vi "FipsAdjacent.vi"() -> (11 "Fips":i32[](array[numeric]))   [LabVIEW 2017] (continued)
, MN\"\t27173\t\"Lyon County, MN\"\t27083\n\"Yellow Medicine County, MN\"\t27173\t\"Redwood County, MN\"\t27127\n\"Yellow Medicine County, MN\"\t27173\t\"Renville County, MN\"\t27129\n\"Yellow Medicine County, MN\"\t27173\t\"Yellow Medicine County, MN\"\t27173\n\"Yellow Medicine County, MN\"\t27173\t\"Deuel County, SD\"\t46039\n\"Adams County, MS\"\t28001\t\"Concordia Parish, LA\"\t22029\n\"Adams County, MS\"\t28001\t\"Tensas Parish, LA\"\t22107\n\"Adams County, MS\"\t28001\t\"Adams County, MS\"\t28001\n\"Adams County, MS\"\t28001\t\"Franklin County, MS\"\t28037\n\"Adams County, MS\"\t28001\t\"Jefferson County, MS\"\t28063\n\"Adams County, MS\"\t28001\t\"Wilkinson County, MS\"\t28157\n\"Alcorn County, MS\"\t28003\t\"Alcorn County, MS\"\t28003\n\"Alcorn County, MS\"\t28003\t\"Prentiss County, MS\"\t28117\n\"Alcorn County, MS\"\t28003\t\"Tippah County, MS\"\t28139\n\"Alcorn County, MS\"\t28003\t\"Tishomingo County, MS\"\t28141\n\"Alcorn County, MS\"\t28003\t\"Hardeman County, TN\"\t47069\n\"Alcorn County, MS\"\t28003\t\"Hardin County, TN\"\t47071\n\"Alcorn County, MS\"\t28003\t\"McNairy County, TN\"\t47109\n\"Amite County, MS\"\t28005\t\"East Feliciana Parish, LA\"\t22037\n\"Amite County, MS\"\t28005\t\"St. Helena Parish, LA\"\t22091\n\"Amite County, MS\"\t28005\t\"Tangipahoa Parish, LA\"\t22105\n\"Amite County, MS\"\t28005\t\"Amite County, MS\"\t28005\n\"Amite County, MS\"\t28005\t\"Franklin County, MS\"\t28037\n\"Amite County, MS\"\t28005\t\"Lincoln County, MS\"\t28085\n\"Amite County, MS\"\t28005\t\"Pike County, MS\"\t28113\n\"Amite County, MS\"\t28005\t\"Wilkinson County, MS\"\t28157\n\"Attala County, MS\"\t28007\t\"Attala County, MS\"\t28007\n\"Attala County, MS\"\t28007\t\"Carroll County, MS\"\t28015\n\"Attala County, MS\"\t28007\t\"Choctaw County, MS\"\t28019\n\"Attala County, MS\"\t28007\t\"Holmes County, MS\"\t28051\n\"Attala County, MS\"\t28007\t\"Leake County, MS\"\t28079\n\"Attala County, MS\"\t28007\t\"Madison County, MS\"\t28089\n\"Attala County, MS\"\t28007\t\"Montgomery County, MS\"\t28097\n\"Attala County, MS\"\t28007\t\"Neshoba County, MS\"\t28099\n\"Attala County, MS\"\t28007\t\"Winston County, MS\"\t28159\n\"Attala County, MS\"\t28007\t\"Yazoo County, MS\"\t28163\n\"Benton County, MS\"\t28009\t\"Benton County, MS\"\t28009\n\"Benton County, MS\"\t28009\t\"Marshall County, MS\"\t28093\n\"Benton County, MS\"\t28009\t\"Tippah County, MS\"\t28139\n\"Benton County, MS\"\t28009\t\"Union County, MS\"\t28145\n\"Benton County, MS\"\t28009\t\"Fayette County, TN\"\t47047\n\"Benton County, MS\"\t28009\t\"Hardeman County, TN\"\t47069\n\"Bolivar County, MS\"\t28011\t\"Chicot County, AR\"\t05017\n\"Bolivar County, MS\"\t28011\t\"Desha County, AR\"\t05041\n\"Bolivar County, MS\"\t28011\t\"Phillips County, AR\"\t05107\n\"Bolivar County, MS\"\t28011\t\"Bolivar County, MS\"\t28011\n\"Bolivar County, MS\"\t28011\t\"Coahoma County, MS\"\t28027\n\"Bolivar County, MS\"\t28011\t\"Sunflower County, MS\"\t28133\n\"Bolivar County, MS\"\t28011\t\"Washington County, MS\"\t28151\n\"Calhoun County, MS\"\t28013\t\"Calhoun County, MS\"\t28013\n\"Calhoun County, MS\"\t28013\t\"Chickasaw County, MS\"\t28017\n\"Calhoun County, MS\"\t28013\t\"Grenada County, MS\"\t28043\n\"Calhoun County, MS\"\t28013\t\"Lafayette County, MS\"\t28071\n\"Calhoun County, MS\"\t28013\t\"Pontotoc County, MS\"\t28115\n\"Calhoun County, MS\"\t28013\t\"Webster County, MS\"\t28155\n\"Calhoun County, MS\"\t28013\t\"Yalobusha County, MS\"\t28161\n\"Carroll County, MS\"\t28015\t\"Attala County, MS\"\t28007\n\"Carroll County, MS\"\t28015\t\"Carroll County, MS\"\t28015\n\"Carroll County, MS\"\t28015\t\"Grenada County, MS\"\t28043\n\"Carroll County, MS\"\t28015\t\"Holmes County, MS\"\t28051\n\"Carroll County, MS\"\t28015\t\"Leflore County, MS\"\t28083\n\"Carroll County, MS\"\t28015\t\"Montgomery County, MS\"\t28097\n\"Chickasaw County, MS\"\t28017\t\"Calhoun County, MS\"\t28013\n\"Chickasaw County, MS\"\t28017\t\"Chickasaw County, MS\"\t28017\n\"Chickasaw County, MS\"\t28017\t\"Clay County, MS\"\t28025\n\"Chickasaw County, MS\"\t28017\t\"Lee County, MS\"\t28081\n\"Chickasaw County, MS\"\t28017\t\"Monroe County, MS\"\t28095\n\"Chickasaw County, MS\"\t28017\t\"Pontotoc County, MS\"\t28115\n\"Chickasaw County, MS\"\t28017\t\"Webster County, MS\"\t28155\n\"Choctaw County, MS\"\t28019\t\"Attala County, MS\"\t28007\n\"Choctaw County, MS\"\t28019\t\"Choctaw County, MS\"\t28019\n\"Choctaw County, MS\"\t28019\t\"Montgomery County, MS\"\t28097\n\"Choctaw County, MS\"\t28019\t\"Oktibbeha County, MS\"\t28105\n\"Choctaw County, MS\"\t28019\t\"Webster County, MS\"\t28155\n\"Choctaw County, MS\"\t28019\t\"Winston County, MS\"\t28159\n\"Claiborne County, MS\"\t28021\t\"Tensas Parish, LA\"\t22107\n\"Claiborne County, MS\"\t28021\t\"Claiborne County, MS\"\t28021\n\"Claiborne County, MS\"\t28021\t\"Copiah County, MS\"\t28029\n\"Claiborne County, MS\"\t28021\t\"Hinds County, MS\"\t28049\n\"Claiborne County, MS\"\t28021\t\"Jefferson County, MS\"\t28063\n\"Claiborne County, MS\"\t28021\t\"Warren County, MS\"\t28149\n\"Clarke County, MS\"\t28023\t\"Choctaw County, AL\"\t01023\n\"Clarke County, MS\"\t28023\t\"Clarke County, MS\"\t28023\n\"Clarke County, MS\"\t28023\t\"Jasper County, MS\"\t28061\n\"Clarke County, MS\"\t28023\t\"Lauderdale County, MS\"\t28075\n\"Clarke County, MS\"\t28023\t\"Newton County, MS\"\t28101\n\"Clarke County, MS\"\t28023\t\"Wayne County, MS\"\t28153\n\"Clay County, MS\"\t28025\t\"Chickasaw County, MS\"\t28017\n\"Clay County, MS\"\t28025\t\"Clay County, MS\"\t28025\n\"Clay County, MS\"\t28025\t\"Lowndes County, MS\"\t28087\n\"Clay County, MS\"\t28025\t\"Monroe County, MS\"\t28095\n\"Clay County, MS\"\t28025\t\"Oktibbeha County, MS\"\t28105\n\"Clay County, MS\"\t28025\t\"Webster County, MS\"\t28155\n\"Coahoma County, MS\"\t28027\t\"Phillips County, AR\"\t05107\n\"Coahoma County, MS\"\t28027\t\"Bolivar County, MS\"\t28011\n\"Coahoma County, MS\"\t28027\t\"Coahoma County, MS\"\t28027\n\"Coahoma County, MS\"\t28027\t\"Quitman County, MS\"\t28119\n\"Coahoma County, MS\"\t28027\t\"Sunflower County, MS\"\t28133\n\"Coahoma County, MS\"\t28027\t\"Tallahatchie County, MS\"\t28135\n\"Coahoma County, MS\"\t28027\t\"Tunica County, MS\"\t28143\n\"Copiah County, MS\"\t28029\t\"Claiborne County, MS\"\t28021\n\"Copiah County, MS\"\t28029\t\"Copiah County, MS\"\t28029\n\"Copiah County, MS\"\t28029\t\"Hinds County, MS\"\t28049\n\"Copiah County, MS\"\t28029\t\"Jefferson County, MS\"\t28063\n\"Copiah County, MS\"\t28029\t\"Lawrence County, MS\"\t28077\n\"Copiah County, MS\"\t28029\t\"Lincoln County, MS\"\t28085\n\"Copiah County, MS\"\t28029\t\"Rankin County, MS\"\t28121\n\"Copiah County, MS\"\t28029\t\"Simpson County, MS\"\t28127\n\"Covington County, MS\"\t28031\t\"Covington County, MS\"\t28031\n\"Covington County, MS\"\t28031\t\"Forrest County, MS\"\t28035\n\"Covington County, MS\"\t28031\t\"Jefferson Davis County, MS\"\t28065\n\"Covington County, MS\"\t28031\t\"Jones County, MS\"\t28067\n\"Covington County, MS\"\t28031\t\"Lamar County, MS\"\t28073\n\"Covington County, MS\"\t28031\t\"Simpson County, MS\"\t28127\n\"Covington County, MS\"\t28031\t\"Smith County, MS\"\t28129\n\"DeSoto County, MS\"\t28033\t\"Crittenden County, AR\"\t05035\n\"DeSoto County, MS\"\t28033\t\"DeSoto County, MS\"\t28033\n\"DeSoto County, MS\"\t28033\t\"Marshall County, MS\"\t28093\n\"DeSoto County, MS\"\t28033\t\"Tate County, MS\"\t28137\n\"DeSoto County, MS\"\t28033\t\"Tunica County, MS\"\t28143\n\"DeSoto County, MS\"\t28033\t\"Shelby County, TN\"\t47157\n\"Forrest County, MS\"\t28035\t\"Covington County, MS\"\t28031\n\"Forrest County, MS\"\t28035\t\"Forrest County, MS\"\t28035\n\"Forrest County, MS\"\t28035\t\"Jones County, MS\"\t28067\n\"Forrest County, MS\"\t28035\t\"Lamar County, MS\"\t28073\n\"Forrest County, MS\"\t28035\t\"Pearl River County, MS\"\t28109\n\"Forrest County, MS\"\t28035\t\"Perry County, MS\"\t28111\n\"Forrest County, MS\"\t28035\t\"Stone County, MS\"\t28131\n\"Franklin County, MS\"\t28037\t\"Adams County, MS\"\t28001\n\"Franklin County, MS\"\t28037\t\"Amite County, MS\"\t28005\n\"Franklin County, MS\"\t28037\t\"Franklin County, MS\"\t28037\n\"Franklin County, MS\"\t28037\t\"Jefferson County, MS\"\t28063\n\"Franklin County, MS\"\t28037\t\"Lincoln County, MS\"\t28085\n\"Franklin County, MS\"\t28037\t\"Wilkinson County, MS\"\t28157\n\"George County, MS\"\t28039\t\"Mobile County, AL\"\t01097\n\"George County, MS\"\t28039\t\"George County, MS\"\t28039\n\"George County, MS\"\t28039\t\"Greene County, MS\"\t28041\n\"George County, MS\"\t28039\t\"Jackson County, MS\"\t28059\n\"George County, MS\"\t28039\t\"Perry County, MS\"\t28111\n\"George County, MS\"\t28039\t\"Stone County, MS\"\t28131\n\"Greene County, MS\"\t28041\t\"Mobile County, AL\"\t01097\n\"Greene County, MS\"\t28041\t\"Washington County, AL\"\t01129\n\"Greene County, MS\"\t28041\t\"George County, MS\"\t28039\n\"Greene County, MS\"\t28041\t\"Greene County, MS\"\t28041\n\"Greene County, MS\"\t28041\t\"Perry County, MS\"\t28111\n\"Greene County, MS\"\t28041\t\"Wayne County, MS\"\t28153\n\"Grenada County, MS\"\t28043\t\"Calhoun County, MS\"\t28013\n\"Grenada County, MS\"\t28043\t\"Carroll County, MS\"\t28015\n\"Grenada County, MS\"\t28043\t\"Grenada County, MS\"\t28043\n\"Grenada County, MS\"\t28043\t\"Leflore County, MS\"\t28083\n\"Grenada County, MS\"\t28043\t\"Montgomery County, MS\"\t28097\n\"Grenada County, MS\"\t28043\t\"Tallahatchie County, MS\"\t28135\n\"Grenada County, MS\"\t28043\t\"Webster County, MS\"\t28155\n\"Grenada County, MS\"\t28043\t\"Yalobusha County, MS\"\t28161\n\"Hancock County, MS\"\t28045\t\"St. Bernard Parish, LA\"\t22087\n\"Hancock County, MS\"\t28045\t\"St. Tammany Parish, LA\"\t22103\n\"Hancock County, MS\"\t28045\t\"Hancock County, MS\"\t28045\n\"Hancock County, MS\"\t28045\t\"Harrison County, MS\"\t28047\n\"Hancock County, MS\"\t28045\t\"Pearl River County, MS\"\t28109\n\"Hancock County, MS\"\t28045\t\"Stone County, MS\"\t28131\n\"Harrison County, MS\"\t28047\t\"St. Bernard Parish, LA\"\t22087\n\"Harrison County, MS\"\t28047\t\"Hancock County, MS\"\t28045\n\"Harrison County, MS\"\t28047\t\"Harrison County, MS\"\t28047\n\"Harrison County, MS\"\t28047\t\"Jackson County, MS\"\t28059\n\"Harrison County, MS\"\t28047\t\"Pearl River County, MS\"\t28109\n\"Harrison County, MS\"\t28047\t\"Stone County, MS\"\t28131\n\"Hinds County, MS\"\t28049\t\"Claiborne County, MS\"\t28021\n\"Hinds County, MS\"\t28049\t\"Copiah County, MS\"\t28029\n\"Hinds County, MS\"\t28049\t\"Hinds County, MS\"\t28049\n\"Hinds County, MS\"\t28049\t\"Madison County, MS\"\t28089\n\"Hinds County, MS\"\t28049\t\"Rankin County, MS\"\t28121\n\"Hinds County, MS\"\t28049\t\"Simpson County, MS\"\t28127\n\"Hinds County, MS\"\t28049\t\"Warren County, MS\"\t28149\n\"Hinds County, MS\"\t28049\t\"Yazoo County, MS\"\t28163\n\"Holmes County, MS\"\t28051\t\"Attala County, MS\"\t28007\n\"Holmes County, MS\"\t28051\t\"Carroll County, MS\"\t28015\n\"Holmes County, MS\"\t28051\t\"Holmes County, MS\"\t28051\n\"Holmes County, MS\"\t28051\t\"Humphreys County, MS\"\t28053\n\"Holmes County, MS\"\t28051\t\"Leflore County, MS\"\t28083\n\"Holmes County, MS\"\t28051\t\"Madison County, MS\"\t28089\n\"Holmes County, MS\"\t28051\t\"Yazoo County, MS\"\t28163\n\"Humphreys County, MS\"\t28053\t\"Holmes County, MS\"\t28051\n\"Humphreys County, MS\"\t28053\t\"Humphreys County, MS\"\t28053\n\"Humphreys County, MS\"\t28053\t\"Leflore County, MS\"\t28083\n\"Humphreys County, MS\"\t28053\t\"Sharkey County, MS\"\t28125\n\"Humphreys County, MS\"\t28053\t\"Sunflower County, MS\"\t28133\n\"Humphreys County, MS\"\t28053\t\"Washington County, MS\"\t28151\n\"Humphreys County, MS\"\t28053\t\"Yazoo County, MS\"\t28163\n\"Issaquena County, MS\"\t28055\t\"Chicot County, AR\"\t05017\n\"Issaquena County, MS\"\t28055\t\"East Carroll Parish, LA\"\t22035\n\"Issaquena County, MS\"\t28055\t\"Issaquena County, MS\"\t28055\n\"Issaquena County, MS\"\t28055\t\"Sharkey County, MS\"\t28125\n\"Issaquena County, MS\"\t28055\t\"Warren County, MS\"\t28149\n\"Issaquena County, MS\"\t28055\t\"Washington County, MS\"\t28151\n\"Issaquena County, MS\"\t28055\t\"Yazoo County, MS\"\t28163\n\"Itawamba County, MS\"\t28057\t\"Franklin County, AL\"\t01059\n\"Itawamba County, MS\"\t28057\t\"Marion County, AL\"\t01093\n\"Itawamba County, MS\"\t28057\t\"Itawamba County, MS\"\t28057\n\"Itawamba County, MS\"\t28057\t\"Lee County, MS\"\t28081\n\"Itawamba County, MS\"\t28057\t\"Monroe County, MS\"\t28095\n\"Itawamba County, MS\"\t28057\t\"Prentiss County, MS\"\t28117\n\"Itawamba County, MS\"\t28057\t\"Tishomingo County, MS\"\t28141\n\"Jackson County, MS\"\t28059\t\"Mobile County, AL\"\t01097\n\"Jackson County, MS\"\t28059\t\"George County, MS\"\t28039\n\"Jackson County, MS\"\t28059\t\"Harrison County, MS\"\t28047\n\"Jackson County, MS\"\t28059\t\"Jackson County, MS\"\t28059\n\"Jackson County, MS\"\t28059\t\"Stone County, MS\"\t28131\n\"Jasper County, MS\"\t28061\t\"Clarke County, MS\"\t28023\n\"Jasper County, MS\"\t28061\t\"Jasper County, MS\"\t28061\n\"Jasper County, MS\"\t28061\t\"Jones County, MS\"\t28067\n\"Jasper County, MS\"\t28061\t\"Lauderdale County, MS\"\t28075\n\"Jasper County, MS\"\t28061\t\"Newton County, MS\"\t28101\n\"Jasper County, MS\"\t28061\t\"Scott County, MS\"\t28123\n\"Jasper County, MS\"\t28061\t\"Smith County, MS\"\t28129\n\"Jasper County, MS\"\t28061\t\"Wayne County, MS\"\t28153\n\"Jefferson County, MS\"\t28063\t\"Tensas Parish, LA\"\t22107\n\"Jefferson County, MS\"\t28063\t\"Adams County, MS\"\t28001\n\"Jefferson County, MS\"\t28063\t\"Claiborne County, MS\"\t28021\n\"Jefferson County, MS\"\t28063\t\"Copiah County, MS\"\t28029\n\"Jefferson County, MS\"\t28063\t\"Franklin County, MS\"\t28037\n\"Jefferson County, MS\"\t28063\t\"Jefferson County, MS\"\t28063\n\"Jefferson County, MS\"\t28063\t\"Lincoln County, MS\"\t28085\n\"Jefferson Davis County, MS\"\t28065\t\"Covington County, MS\"\t28031\n\"Jefferson Davis County, MS\"\t28065\t\"Jefferson Davis County, MS\"\t28065\n\"Jefferson Davis County, MS\"\t28065\t\"Lamar County, MS\"\t28073\n\"Jefferson Davis County, MS\"\t28065\t\"Lawrence County, MS\"\t28077\n\"Jefferson Davis County, MS\"\t28065\t\"Marion County, MS\"\t28091\n\"Jefferson Davis County, MS\"\t28065\t\"Simpson County, MS\"\t28127\n\"Jones County, MS\"\t28067\t\"Covington County, MS\"\t28031\n\"Jones County, MS\"\t28067\t\"Forrest County, MS\"\t28035\n\"Jones County, MS\"\t28067\t\"Jasper County, MS\"\t28061\n\"Jones County, MS\"\t28067\t\"Jones County, MS\"\t28067\n\"Jones County, MS\"\t28067\t\"Perry County, MS\"\t28111\n\"Jones County, MS\"\t28067\t\"Smith County, MS\"\t28129\n\"Jones County, MS\"\t28067\t\"Wayne County, MS\"\t28153\n\"Kemper County, MS\"\t28069\t\"Sumter County, AL\"\t01119\n\"Kemper County, MS\"\t28069\t\"Kemper County, MS\"\t28069\n\"Kemper County, MS\"\t28069\t\"Lauderdale County, MS\"\t28075\n\"Kemper County, MS\"\t28069\t\"Neshoba County, MS\"\t28099\n\"Kemper County, MS\"\t28069\t\"Newton County, MS\"\t28101\n\"Kemper County, MS\"\t28069\t\"Noxubee County, MS\"\t28103\n\"Kemper County, MS\"\t28069\t\"Winston County, MS\"\t28159\n\"Lafayette County, MS\"\t28071\t\"Calhoun County, MS\"\t28013\n\"Lafayette County, MS\"\t28071\t\"Lafayette County, MS\"\t28071\n\"Lafayette County, MS\"\t28071\t\"Marshall County, MS\"\t28093\n\"Lafayette County, MS\"\t28071\t\"Panola County, MS\"\t28107\n\"Lafayette County, MS\"\t28071\t\"Pontotoc County, MS\"\t28115\n\"Lafayette County, MS\"\t28071\t\"Tate County, MS\"\t28137\n\"Lafayette County, MS\"\t28071\t\"Union County, MS\"\t28145\n\"Lafayette County, MS\"\t28071\t\"Yalobusha County, MS\"\t28161\n\"Lamar County, MS\"\t28073\t\"Covington County, MS\"\t28031\n\"Lamar County, MS\"\t28073\t\"Forrest County, MS\"\t28035\n\"Lamar County, MS\"\t28073\t\"Jefferson Davis County, MS\"\t28065\n\"Lamar County, MS\"\t28073\t\"Lamar County, MS\"\t28073\n\"Lamar County, MS\"\t28073\t\"Marion County, MS\"\t28091\n\"Lamar County, MS\"\t28073\t\"Pearl River County, MS\"\t28109\n\"Lauderdale County, MS\"\t28075\t\"Choctaw County, AL\"\t01023\n\"Lauderdale County, MS\"\t28075\t\"Sumter County, AL\"\t01119\n\"Lauderdale County, MS\"\t28075\t\"Clarke County, MS\"\t28023\n\"Lauderdale County, MS\"\t28075\t\"Jasper County, MS\"\t28061\n\"Lauderdale County, MS\"\t28075\t\"Kemper County, MS\"\t28069\n\"Lauderdale County, MS\"\t28075\t\"Lauderdale County, MS\"\t28075\n\"Lauderdale County, MS\"\t28075\t\"Neshoba County, MS\"\t28099\n\"Lauderdale County, MS\"\t28075\t\"Newton County, MS\"\t28101\n\"Lawrence County, MS\"\t28077\t\"Copiah County, MS\"\t28029\n\"Lawrence County, MS\"\t28077\t\"Jefferson Davis County, MS\"\t28065\n\"Lawrence County, MS\"\t28077\t\"Lawrence County, MS\"\t28077\n\"Lawrence County, MS\"\t28077\t\"Lincoln County, MS\"\t28085\n\"Lawrence County, MS\"\t28077\t\"Marion County, MS\"\t28091\n\"Lawrence County, MS\"\t28077\t\"Simpson County, MS\"\t28127\n\"Lawrence County, MS\"\t28077\t\"Walthall County, MS\"\t28147\n\"Leake County, MS\"\t28079\t\"Attala County, MS\"\t28007\n\"Leake County, MS\"\t28079\t\"Leake County, MS\"\t28079\n\"Leake County, MS\"\t28079\t\"Madison County, MS\"\t28089\n\"Leake County, MS\"\t28079\t\"Neshoba County, MS\"\t28099\n\"Leake County, MS\"\t28079\t\"Newton County, MS\"\t28101\n\"Leake County, MS\"\t28079\t\"Scott County, MS\"\t28123\n\"Leake County, MS\"\t28079\t\"Winston County, MS\"\t28159\n\"Lee County, MS\"\t28081\t\"Chickasaw County, MS\"\t28017\n\"Lee County, MS\"\t28081\t\"Itawamba County, MS\"\t28057\n\"Lee County, MS\"\t28081\t\"Lee County, MS\"\t28081\n\"Lee County, MS\"\t28081\t\"Monroe County, MS\"\t28095\n\"Lee County, MS\"\t28081\t\"Pontotoc County, MS\"\t28115\n\"Lee County, MS\"\t28081\t\"Prentiss County, MS\"\t28117\n\"Lee County, MS\"\t28081\t\"Union County, MS\"\t28145\n\"Leflore County, MS\"\t28083\t\"Carroll County, MS\"\t28015\n\"Leflore County, MS\"\t28083\t\"Grenada County, MS\"\t28043\n\"Leflore County, MS\"\t28083\t\"Holmes County, MS\"\t28051\n\"Leflore County, MS\"\t28083\t\"Humphreys County, MS\"\t28053\n\"Leflore County, MS\"\t28083\t\"Leflore County, MS\"\t28083\n\"Leflore County, MS\"\t28083\t\"Sunflower County, MS\"\t28133\n\"Leflore County, MS\"\t28083\t\"Tallahatchie County, MS\"\t28135\n\"Lincoln County, MS\"\t28085\t\"Amite County, MS\"\t28005\n\"Lincoln County, MS\"\t28085\t\"Copiah County, MS\"\t28029\n\"Lincoln County, MS\"\t28085\t\"Franklin County, MS\"\t28037\n\"Lincoln County, MS\"\t28085\t\"Jefferson County, MS\"\t28063\n\"Lincoln County, MS\"\t28085\t\"Lawrence County, MS\"\t28077\n\"Lincoln County, MS\"\t28085\t\"Lincoln County, MS\"\t28085\n\"Lincoln County, MS\"\t28085\t\"Pike County, MS\"\t28113\n\"Lincoln County, MS\"\t28085\t\"Walthall County, MS\"\t28147\n\"Lowndes County, MS\"\t28087\t\"Lamar County, AL\"\t01075\n\"Lowndes County, MS\"\t28087\t\"Pickens County, AL\"\t01107\n\"Lowndes County, MS\"\t28087\t\"Clay County, MS\"\t28025\n\"Lowndes County, MS\"\t28087\t\"Lowndes County, MS\"\t28087\n\"Lowndes County, MS\"\t28087\t\"Monroe County, MS\"\t28095\n\"Lowndes County, MS\"\t28087\t\"Noxubee County, MS\"\t28103\n\"Lowndes County, MS\"\t28087\t\"Oktibbeha County, MS\"\t28105\n\"Madison County, MS\"\t28089\t\"Attala County, MS\"\t28007\n\"Madison County, MS\"\t28089\t\"Hinds County, MS\"\t28049\n\"Madison County, MS\"\t28089\t\"Holmes County, MS\"\t28051\n\"Madison County, MS\"\t28089\t\"Leake County, MS\"\t28079\n\"Madison County, MS\"\t28089\t\"Madison County, MS\"\t28089\n\"Madison County, MS\"\t28089\t\"Rankin County, MS\"\t28121\n\"Madison County, MS\"\t28089\t\"Scott County, MS\"\t28123\n\"Madison County, MS\"\t28089\t\"Yazoo County, MS\"\t28163\n\"Marion County, MS\"\t28091\t\"Washington Parish, LA\"\t22117\n\"Marion County, MS\"\t28091\t\"Jefferson Davis County, MS\"\t28065\n\"Marion County, MS\"\t28091\t\"Lamar County, MS\"\t28073\n\"Marion County, MS\"\t28091\t\"Lawrence County, MS\"\t28077\n\"Marion County, MS\"\t28091\t\"Marion County, MS\"\t28091\n\"Marion County, MS\"\t28091\t\"Pearl River County, MS\"\t28109\n\"Marion County, MS\"\t28091\t\"Walthall County, MS\"\t28147\n\"Marshall County, MS\"\t28093\t\"Benton County, MS\"\t28009\n\"Marshall County, MS\"\t28093\t\"DeSoto County, MS\"\t28033\n\"Marshall County, MS\"\t28093\t\"Lafayette County, MS\"\t28071\n\"Marshall County, MS\"\t28093\t\"Marshall County, MS\"\t28093\n\"Marshall County, MS\"\t28093\t\"Tate County, MS\"\t28137\n\"Marshall County, MS\"\t28093\t\"Union County, MS\"\t28145\n\"Marshall County, MS\"\t28093\t\"Fayette County, TN\"\t47047\n\"Marshall County, MS\"\t28093\t\"Shelby County, TN\"\t47157\n\"Monroe County, MS\"\t28095\t\"Lamar County, AL\"\t01075\n\"Monroe County, MS\"\t28095\t\"Marion County, AL\"\t01093\n\"Monroe County, MS\"\t28095\t\"Chickasaw County, MS\"\t28017\n\"Monroe County, MS\"\t28095\t\"Clay County, MS\"\t28025\n\"Monroe County, MS\"\t28095\t\"Itawamba County, MS\"\t28057\n\"Monroe County, MS\"\t28095\t\"Lee County, MS\"\t28081\n\"Monroe County, MS\"\t28095\t\"Lowndes County, MS\"\t28087\n\"Monroe County, MS\"\t28095\t\"Monroe County, MS\"\t28095\n\"Montgomery County, MS\"\t28097\t\"Attala County, MS\"\t28007\n\"Montgomery County, MS\"\t28097\t\"Carroll County, MS\"\t28015\n\"Montgomery County, MS\"\t28097\t\"Choctaw County, MS\"\t28019\n\"Montgomery County, MS\"\t28097\t\"Grenada County, MS\"\t28043\n\"Montgomery County, MS\"\t28097\t\"Montgomery County, MS\"\t28097\n\"Montgomery County, MS\"\t28097\t\"Webster County, MS\"\t28155\n\"Neshoba County, MS\"\t28099\t\"Attala County, MS\"\t28007\n\"Neshoba County, MS\"\t28099\t\"Kemper County, MS\"\t28069\n\"Neshoba County, MS\"\t28099\t\"Lauderdale County, MS\"\t28075\n\"Neshoba County, MS\"\t28099\t\"Leake County, MS\"\t28079\n\"Neshoba County, MS\"\t28099\t\"Neshoba County, MS\"\t28099\n\"Neshoba County, MS\"\t28099\t\"Newton County, MS\"\t28101\n\"Neshoba County, MS\"\t28099\t\"Winston County, MS\"\t28159\n\"Newton County, MS\"\t28101\t\"Clarke County, MS\"\t28023\n\"Newton County, MS\"\t28101\t\"Jasper County, MS\"\t28061\n\"Newton County, MS\"\t28101\t\"Kemper County, MS\"\t28069\n\"Newton County, MS\"\t28101\t\"Lauderdale County, MS\"\t28075\n\"Newton County, MS\"\t28101\t\"Leake County, MS\"\t28079\n\"Newton County, MS\"\t28101\t\"Neshoba County, MS\"\t28099\n\"Newton County, MS\"\t28101\t\"Newton County, MS\"\t28101\n\"Newton County, MS\"\t28101\t\"Scott County, MS\"\t28123\n\"Newton County, MS\"\t28101\t\"Smith County, MS\"\t28129\n\"Noxubee County, MS\"\t28103\t\"Pickens County, AL\"\t01107\n\"Noxubee County, MS\"\t28103\t\"Sumter County, AL\"\t01119\n\"Noxubee County, MS\"\t28103\t\"Kemper County, MS\"\t28069\n\"Noxubee County, MS\"\t28103\t\"Lowndes County, MS\"\t28087\n\"Noxubee County, MS\"\t28103\t\"Noxubee County, MS\"\t28103\n\"Noxubee County, MS\"\t28103\t\"Oktibbeha County, MS\"\t28105\n\"Noxubee County, MS\"\t28103\t\"Winston County, MS\"\t28159\n\"Oktibbeha County, MS\"\t28105\t\"Choctaw County, MS\"\t28019\n\"Oktibbeha County, MS\"\t28105\t\"Clay County, MS\"\t28025\n\"Oktibbeha County, MS\"\t28105\t\"Lowndes County, MS\"\t28087\n\"Oktibbeha County, MS\"\t28105\t\"Noxubee County, MS\"\t28103\n\"Oktibbeha County, MS\"\t28105\t\"Oktibbeha County, MS\"\t28105\n\"Oktibbeha County, MS\"\t28105\t\"Webster County, MS\"\t28155\n\"Oktibbeha County, MS\"\t28105\t\"Winston County, MS\"\t28159\n\"Panola County, MS\"\t28107\t\"Lafayette County, MS\"\t28071\n\"Panola County, MS\"\t28107\t\"Panola County, MS\"\t28107\n\"Panola County, MS\"\t28107\t\"Quitman County, MS\"\t28119\n\"Panola County, MS\"\t28107\t\"Tallahatchie County, MS\"\t28135\n\"Panola County, MS\"\t28107\t\"Tate County, MS\"\t28137\n\"Panola County, MS\"\t28107\t\"Tunica County, MS\"\t28143\n\"Panola County, MS\"\t28107\t\"Yalobusha County, MS\"\t28161\n\"Pearl River County, MS\"\t28109\t\"St. Tammany Parish, LA\"\t22103\n\"Pearl River County, MS\"\t28109\t\"Washington Parish, LA\"\t22117\n\"Pearl River County, MS\"\t28109\t\"Forrest County, MS\"\t28035\n\"Pearl River County, MS\"\t28109\t\"Hancock County, MS\"\t28045\n\"Pearl River County, MS\"\t28109\t\"Harrison County, MS\"\t28047\n\"Pearl River County, MS\"\t28109\t\"Lamar County, MS\"\t28073\n\"Pearl River County, MS\"\t28109\t\"Marion County, MS\"\t28091\n\"Pearl River County, MS\"\t28109\t\"Pearl River County, MS\"\t28109\n\"Pearl River County, MS\"\t28109\t\"Stone County, MS\"\t28131\n\"Perry County, MS\"\t28111\t\"Forrest County, MS\"\t28035\n\"Perry County, MS\"\t28111\t\"George County, MS\"\t28039\n\"Perry County, MS\"\t28111\t\"Greene County, MS\"\t28041\n\"Perry County, MS\"\t28111\t\"Jones County, MS\"\t28067\n\"Perry County, MS\"\t28111\t\"Perry County, MS\"\t28111\n\"Perry County, MS\"\t28111\t\"Stone County, MS\"\t28131\n\"Perry County, MS\"\t28111\t\"Wayne County, MS\"\t28153\n\"Pike County, MS\"\t28113\t\"Tangipahoa Parish, LA\"\t22105\n\"Pike County, MS\"\t28113\t\"Washington Parish, LA\"\t22117\n\"Pike County, MS\"\t28113\t\"Amite County, MS\"\t28005\n\"Pike County, MS\"\t28113\t\"Lincoln County, MS\"\t28085\n\"Pike County, MS\"\t28113\t\"Pike County, MS\"\t28113\n\"Pike County, MS\"\t28113\t\"Walthall County, MS\"\t28147\n\"Pontotoc County, MS\"\t28115\t\"Calhoun County, MS\"\t28013\n\"Pontotoc County, MS\"\t28115\t\"Chickasaw County, MS\"\t28017\n\"Pontotoc County, MS\"\t28115\t\"Lafayette County, MS\"\t28071\n\"Pontotoc County, MS\"\t28115\t\"Lee County, MS\"\t28081\n\"Pontotoc County, MS\"\t28115\t\"Pontotoc County, MS\"\t28115\n\"Pontotoc County, MS\"\t28115\t\"Union County, MS\"\t28145\n\"Prentiss County, MS\"\t28117\t\"Alcorn County, MS\"\t28003\n\"Prentiss County, MS\"\t28117\t\"Itawamba County, MS\"\t28057\n\"Prentiss County, MS\"\t28117\t\"Lee County, MS\"\t28081\n\"Prentiss County, MS\"\t28117\t\"Prentiss County, MS\"\t28117\n\"Prentiss County, MS\"\t28117\t\"Tippah County, MS\"\t28139\n\"Prentiss County, MS\"\t28117\t\"Tishomingo County, MS\"\t28141\n\"Prentiss County, MS\"\t28117\t\"Union County, MS\"\t28145\n\"Quitman County, MS\"\t28119\t\"Coahoma County, MS\"\t28027\n\"Quitman County, MS\"\t28119\t\"Panola County, MS\"\t28107\n\"Quitman County, MS\"\t28119\t\"Quitman County, MS\"\t28119\n\"Quitman County, MS\"\t28119\t\"Tallahatchie County, MS\"\t28135\n\"Quitman County, MS\"\t28119\t\"Tunica County, MS\"\t28143\n\"Rankin County, MS\"\t28121\t\"Copiah County, MS\"\t28029\n\"Rankin County, MS\"\t28121\t\"Hinds County, MS\"\t28049\n\"Rankin County, MS\"\t28121\t\"Madison County, MS\"\t28089\n\"Rankin County, MS\"\t28121\t\"Rankin County, MS\"\t28121\n\"Rankin County, MS\"\t28121\t\"Scott County, MS\"\t28123\n\"Rankin County, MS\"\t28121\t\"Simpson County, MS\"\t28127\n\"Rankin County, MS\"\t28121\t\"Smith County, MS\"\t28129\n\"Scott County, MS\"\t28123\t\"Jasper County, MS\"\t28061\n\"Scott County, MS\"\t28123\t\"Leake County, MS\"\t28079\n\"Scott County, MS\"\t28123\t\"Madison County, MS\"\t28089\n\"Scott County, MS\"\t28123\t\"Newton County, MS\"\t28101\n\"Scott County, MS\"\t28123\t\"Rankin County, MS\"\t28121\n\"Scott County, MS\"\t28123\t\"Scott County, MS\"\t28123\n\"Scott County, MS\"\t28123\t\"Smith County, MS\"\t28129\n\"Sharkey County, MS\"\t28125\t\"Humphreys County, MS\"\t28053\n\"Sharkey County, MS\"\t28125\t\"Issaquena County, MS\"\t28055\n\"Sharkey County, MS\"\t28125\t\"Sharkey County, MS\"\t28125\n\"Sharkey County, MS\"\t28125\t\"Washington County, MS\"\t28151\n\"Sharkey County, MS\"\t28125\t\"Yazoo County, MS\"\t28163\n\"Simpson County, MS\"\t28127\t\"Copiah County, MS\"\t28029\n\"Simpson County, MS\"\t28127\t\"Covington County, MS\"\t28031\n\"Simpson County, MS\"\t28127\t\"Hinds County, MS\"\t28049\n\"Simpson County, MS\"\t28127\t\"Jefferson Davis County, MS\"\t28065\n\"Simpson County, MS\"\t28127\t\"Lawrence County, MS\"\t28077\n\"Simpson County, MS\"\t28127\t\"Rankin County, MS\"\t28121\n\"Simpson County, MS\"\t28127\t\"Simpson County, MS\"\t28127\n\"Simpson County, MS\"\t28127\t\"Smith County, MS\"\t28129\n\"Smith County, MS\"\t28129\t\"Covington County, MS\"\t28031\n\"Smith County, MS\"\t28129\t\"Jasper County, MS\"\t28061\n\"Smith County, MS\"\t28129\t\"Jones County, MS\"\t28067\n\"Smith County, MS\"\t28129\t\"Newton County, MS\"\t28101\n\"Smith County, MS\"\t28129\t\"Rankin County, MS\"\t28121\n\"Smith County, MS\"\t28129\t\"Scott County, MS\"\t28123\n\"Smith County, MS\"\t28129\t\"Simpson County, MS\"\t28127\n\"Smith County, MS\"\t28129\t\"Smith County, MS\"\t28129\n\"Stone County, MS\"\t28131\t\"Forrest County, MS\"\t28035\n\"Stone County, MS\"\t28131\t\"George County, MS\"\t28039\n\"Stone County, MS\"\t28131\t\"Hancock County, MS\"\t28045\n\"Stone County, MS\"\t28131\t\"Harrison County, MS\"\t28047\n\"Stone County, MS\"\t28131\t\"Jackson County, MS\"\t28059\n\"Stone County, MS\"\t28131\t\"Pearl River County, MS\"\t28109\n\"Stone County, MS\"\t28131\t\"Perry County, MS\"\t28111\n\"Stone County, MS\"\t28131\t\"Stone County, MS\"\t28131\n\"Sunflower County, MS\"\t28133\t\"Bolivar County, MS\"\t28011\n\"Sunflower County, MS\"\t28133\t\"Coahoma County, MS\"\t28027\n\"Sunflower County, MS\"\t28133\t\"Humphreys County, MS\"\t28053\n\"Sunflower County, MS\"\t28133\t\"Leflore County, MS\"\t28083\n\"Sunflower County, MS\"\t28133\t\"Sunflower County, MS\"\t28133\n\"Sunflower County, MS\"\t28133\t\"Tallahatchie County, MS\"\t28135\n\"Sunflower County, MS\"\t28133\t\"Washington County, MS\"\t28151\n\"Tallahatchie County, MS\"\t28135\t\"Coahoma County, MS\"\t28027\n\"Tallahatchie County, MS\"\t28135\t\"Grenada County, MS\"\t28043\n\"Tallahatchie County, MS\"\t28135\t\"Leflore County, MS\"\t28083\n\"Tallahatchie County, MS\"\t28135\t\"Panola County, MS\"\t28107\n\"Tallahatchie County, MS\"\t28135\t\"Quitman County, MS\"\t28119\n\"Tallahatchie County, MS\"\t28135\t\"Sunflower County, MS\"\t28133\n\"Tallahatchie County, MS\"\t28135\t\"Tallahatchie County, MS\"\t28135\n\"Tallahatchie County, MS\"\t28135\t\"Yalobusha County, MS\"\t28161\n\"Tate County, MS\"\t28137\t\"DeSoto County, MS\"\t28033\n\"Tate County, MS\"\t28137\t\"Lafayette County, MS\"\t28071\n\"Tate County, MS\"\t28137\t\"Marshall County, MS\"\t28093\n\"Tate County, MS\"\t28137\t\"Panola County, MS\"\t28107\n\"Tate County, MS\"\t28137\t\"Tate County, MS\"\t28137\n\"Tate County, MS\"\t28137\t\"Tunica County, MS\"\t28143\n\"Tippah County, MS\"\t28139\t\"Alcorn County, MS\"\t28003\n\"Tippah County, MS\"\t28139\t\"Benton County, MS\"\t28009\n\"Tippah County, MS\"\t28139\t\"Prentiss County, MS\"\t28117\n\"Tippah County, MS\"\t28139\t\"Tippah County, MS\"\t28139\n\"Tippah County, MS\"\t28139\t\"Union County, MS\"\t28145\n\"Tippah County, MS\"\t28139\t\"Hardeman County, TN\"\t47069\n\"Tishomingo County, MS\"\t28141\t\"Colbert County, AL\"\t01033\n\"Tishomingo County, MS\"\t28141\t\"Franklin County, AL\"\t01059\n\"Tishomingo County, MS\"\t28141\t\"Lauderdale County, AL\"\t01077\n\"Tishomingo County, MS\"\t28141\t\"Alcorn County, MS\"\t28003\n\"Tishomingo County, MS\"\t28141\t\"Itawamba County, MS\"\t28057\n\"Tishomingo County, MS\"\t28141\t\"Prentiss County, MS\"\t28117\n\"Tishomingo County, MS\"\t28141\t\"Tishomingo County, MS\"\t28141\n\"Tishomingo County, MS\"\t28141\t\"Hardin County, TN\"\t47071\n\"Tunica County, MS\"\t28143\t\"Crittenden County, AR\"\t05035\n\"Tunica County, MS\"\t28143\t\"Lee County, AR\"\t05077\n\"Tunica County, MS\"\t28143\t\"Phillips County, AR\"\t05107\n\"Tunica County, MS\"\t28143\t\"Coahoma County, MS\"\t28027\n\"Tunica County, MS\"\t28143\t\"DeSoto County, MS\"\t28033\n\"Tunica County, MS\"\t28143\t\"Panola County, MS\"\t28107\n\"Tunica County, MS\"\t28143\t\"Quitman County, MS\"\t28119\n\"Tunica County, MS\"\t28143\t\"Tate County, MS\"\t28137\n\"Tunica County, MS\"\t28143\t\"Tunica County, MS\"\t28143\n\"Union County, MS\"\t28145\t\"Benton County, MS\"\t28009\n\"Union County, MS\"\t28145\t\"Lafayette County, MS\"\t28071\n\"Union County, MS\"\t28145\t\"Lee County, MS\"\t28081\n\"Union County, MS\"\t28145\t\"Marshall County, MS\"\t28093\n\"Union County, MS\"\t28145\t\"Pontotoc County, MS\"\t28115\n\"Union County, MS\"\t28145\t\"Prentiss County, MS\"\t28117\n\"Union County, MS\"\t28145\t\"Tippah County, MS\"\t28139\n\"Union County, MS\"\t28145\t\"Union County, MS\"\t28145\n\"Walthall County, MS\"\t28147\t\"Washington Parish, LA\"\t22117\n\"Walthall County, MS\"\t28147\t\"Lawrence County, MS\"\t28077\n\"Walthall County, MS\"\t28147\t\"Lincoln County, MS\"\t28085\n\"Walthall County, MS\"\t28147\t\"Marion County, MS\"\t28091\n\"Walthall County, MS\"\t28147\t\"Pike County, MS\"\t28113\n\"Walthall County, MS\"\t28147\t\"Walthall County, MS\"\t28147\n\"Warren County, MS\"\t28149\t\"East Carroll Parish, LA\"\t22035\n\"Warren County, MS\"\t28149\t\"Madison Parish, LA\"\t22065\n\"Warren County, MS\"\t28149\t\"Tensas Parish, LA\"\t22107\n\"Warren County, MS\"\t28149\t\"Claiborne County, MS\"\t28021\n\"Warren County, MS\"\t28149\t\"Hinds County, MS\"\t28049\n\"Warren County, MS\"\t28149\t\"Issaquena County, MS\"\t28055\n\"Warren County, MS\"\t28149\t\"Warren County, MS\"\t28149\n\"Warren County, MS\"\t28149\t\"Yazoo County, MS\"\t28163\n\"Washington County, MS\"\t28151\t\"Chicot County, AR\"\t05017\n\"Washington County, MS\"\t28151\t\"Bolivar County, MS\"\t28011\n\"Washington County, MS\"\t28151\t\"Humphreys County, MS\"\t28053\n\"Washington County, MS\"\t28151\t\"Issaquena County, MS\"\t28055\n\"Washington County, MS\"\t28151\t\"Sharkey County, MS\"\t28125\n\"Washington County, MS\"\t28151\t\"Sunflower County, MS\"\t28133\n\"Washington County, MS\"\t28151\t\"Washington County, MS\"\t28151\n\"Wayne County, MS\"\t28153\t\"Choctaw County, AL\"\t01023\n\"Wayne County, MS\"\t28153\t\"Washington County, AL\"\t01129\n\"Wayne County, MS\"\t28153\t\"Clarke County, MS\"\t28023\n\"Wayne County, MS\"\t28153\t\"Greene County, MS\"\t28041\n\"Wayne County, MS\"\t28153\t\"Jasper County, MS\"\t28061\n\"Wayne County, MS\"\t28153\t\"Jones County, MS\"\t28067\n\"Wayne County, MS\"\t28153\t\"Perry County, MS\"\t28111\n\"Wayne County, MS\"\t28153\t\"Wayne County, MS\"\t28153\n\"Webster County, MS\"\t28155\t\"Calhoun County, MS\"\t28013\n\"Webster County, MS\"\t28155\t\"Chickasaw County, MS\"\t28017\n\"Webster County, MS\"\t28155\t\"Choctaw County, MS\"\t28019\n\"Webster County, MS\"\t28155\t\"Clay County, MS\"\t28025\n\"Webster County, MS\"\t28155\t\"Grenada County, MS\"\t28043\n\"Webster County, MS\"\t28155\t\"Montgomery County, MS\"\t28097\n\"Webster County, MS\"\t28155\t\"Oktibbeha County, MS\"\t28105\n\"Webster County, MS\"\t28155\t\"Webster County, MS\"\t28155\n\"Wilkinson County, MS\"\t28157\t\"Concordia Parish, LA\"\t22029\n\"Wilkinson County, MS\"\t28157\t\"East Feliciana Parish, LA\"\t22037\n\"Wilkinson County, MS\"\t28157\t\"West Feliciana Parish, LA\"\t22125\n\"Wilkinson County, MS\"\t28157\t\"Adams County, MS\"\t28001\n\"Wilkinson County, MS\"\t28157\t\"Amite County, MS\"\t28005\n\"Wilkinson County, MS\"\t28157\t\"Franklin County, MS\"\t28037\n\"Wilkinson County, MS\"\t28157\t\"Wilkinson County, MS\"\t28157\n\"Winston County, MS\"\t28159\t\"Attala County, MS\"\t28007\n\"Winston County, MS\"\t28159\t\"Choctaw County, MS\"\t28019\n\"Winston County, MS\"\t28159\t\"Kemper County, MS\"\t28069\n\"Winston County, MS\"\t28159\t\"Leake County, MS\"\t28079\n\"Winston County, MS\"\t28159\t\"Neshoba County, MS\"\t28099\n\"Winston County, MS\"\t28159\t\"Noxubee County, MS\"\t28103\n\"Winston County, MS\"\t28159\t\"Oktibbeha County, MS\"\t28105\n\"Winston County, MS\"\t28159\t\"Winston County, MS\"\t28159\n\"Yalobusha County, MS\"\t28161\t\"Calhoun County, MS\"\t28013\n\"Yalobusha County, MS\"\t28161\t\"Grenada County, MS\"\t28043\n\"Yalobusha County, MS\"\t28161\t\"Lafayette County, MS\"\t28071\n\"Yalobusha County, MS\"\t28161\t\"Panola County, MS\"\t28107\n\"Yalobusha County, MS\"\t28161\t\"Tallahatchie County, MS\"\t28135\n\"Yalobusha County, MS\"\t28161\t\"Yalobusha County, MS\"\t28161\n\"Yazoo County, MS\"\t28163\t\"Attala County, MS\"\t28007\n\"Yazoo County, MS\"\t28163\t\"Hinds County, MS\"\t28049\n\"Yazoo County, MS\"\t28163\t\"Holmes County, MS\"\t28051\n\"Yazoo County, MS\"\t28163\t\"Humphreys County, MS\"\t28053\n\"Yazoo County, MS\"\t28163\t\"Issaquena County, MS\"\t28055\n\"Yazoo County, MS\"\t28163\t\"Madison County, MS\"\t28089\n\"Yazoo County, MS\"\t28163\t\"Sharkey County, MS\"\t28125\n\"Yazoo County, MS\"\t28163\t\"Warren County, MS\"\t28149\n\"Yazoo County, MS\"\t28163\t\"Yazoo County, MS\"\t28163\n\"Adair County, MO\"\t29001\t\"Adair County, MO\"\t29001\n\"Adair County, MO\"\t29001\t\"Knox County, MO\"\t29103\n\"Adair County, MO\"\t29001\t\"Linn County, MO\"\t29115\n\"Adair County, MO\"\t29001\t\"Macon County, MO\"\t29121\n\"Adair County, MO\"\t29001\t\"Putnam County, MO\"\t29171\n\"Adair County, MO\"\t29001\t\"Schuyler County, MO\"\t29197\n\"Adair County, MO\"\t29001\t\"Scotland County, MO\"\t29199\n\"Adair County, MO\"\t29001\t\"Sullivan County, MO\"\t29211\n\"Andrew County, MO\"\t29003\t\"Doniphan County, KS\"\t20043\n\"Andrew County, MO\"\t29003\t\"Andrew County, MO\"\t29003\n\"Andrew County, MO\"\t29003\t\"Buchanan County, MO\"\t29021\n\"Andrew County, MO\"\t29003\t\"DeKalb County, MO\"\t29063\n\"Andrew County, MO\"\t29003\t\"Gentry County, MO\"\t29075\n\"Andrew County, MO\"\t29003\t\"Holt County, MO\"\t29087\n\"Andrew County, MO\"\t29003\t\"Nodaway County, MO\"\t29147\n\"Atchison County, MO\"\t29005\t\"Fremont County, IA\"\t19071\n\"Atchison County, MO\"\t29005\t\"Page County, IA\"\t19145\n\"Atchison County, MO\"\t29005\t\"Atchison County, MO\"\t29005\n\"Atchison County, MO\"\t29005\t\"Holt County, MO\"\t29087\n\"Atchison County, MO\"\t29005\t\"Nodaway County, MO\"\t29147\n\"Atchison County, MO\"\t29005\t\"Nemaha County, NE\"\t31127\n\"Atchison County, MO\"\t29005\t\"Otoe County, NE\"\t31131\n\"Audrain County, MO\"\t29007\t\"Audrain County, MO\"\t29007\n\"Audrain County, MO\"\t29007\t\"Boone County, MO\"\t29019\n\"Audrain County, MO\"\t29007\t\"Callaway County, MO\"\t29027\n\"Audrain County, MO\"\t29007\t\"Monroe County, MO\"\t29137\n\"Audrain County, MO\"\t29007\t\"Montgomery County, MO\"\t29139\n\"Audrain County, MO\"\t29007\t\"Pike County, MO\"\t29163\n\"Audrain County, MO\"\t29007\t\"Ralls County, MO\"\t29173\n\"Audrain County, MO\"\t29007\t\"Randolph County, MO\"\t29175\n\"Barry County, MO\"\t29009\t\"Benton County, AR\"\t05007\n\"Barry County, MO\"\t29009\t\"Carroll County, AR\"\t05015\n\"Barry County, MO\"\t29009\t\"Barry County, MO\"\t29009\n\"Barry County, MO\"\t29009\t\"Lawrence County, MO\"\t29109\n\"Barry County, MO\"\t29009\t\"McDonald County, MO\"\t29119\n\"Barry County, MO\"\t29009\t\"Newton County, MO\"\t29145\n\"Barry County, MO\"\t29009\t\"Stone County, MO\"\t29209\n\"Barton County, MO\"\t29011\t\"Crawford County, KS\"\t20037\n\"Barton County, MO\"\t29011\t\"Barton County, MO\"\t29011\n\"Barton County, MO\"\t29011\t\"Cedar County, MO\"\t29039\n\"Barton County, MO\"\t29011\t\"Dade County, MO\"\t29057\n\"Barton County, MO\"\t29011\t\"Jasper County, MO\"\t29097\n\"Barton County, MO\"\t29011\t\"Vernon County, MO\"\t29217\n\"Bates County, MO\"\t29013\t\"Linn County, KS\"\t20107\n\"Bates County, MO\"\t29013\t\"Miami County, KS\"\t20121\n\"Bates County, MO\"\t29013\t\"Bates County, MO\"\t29013\n\"Bates County, MO\"\t29013\t\"Cass County, MO\"\t29037\n\"Bates County, MO\"\t29013\t\"Henry County, MO\"\t29083\n\"Bates County, MO\"\t29013\t\"St. Clair County, MO\"\t29185\n\"Bates County, MO\"\t29013\t\"Vernon County, MO\"\t29217\n\"Benton County, MO\"\t29015\t\"Benton County, MO\"\t29015\n\"Benton County, MO\"\t29015\t\"Camden County, MO\"\t29029\n\"Benton County, MO\"\t29015\t\"Henry County, MO\"\t29083\n\"Benton County, MO\"\t29015\t\"Hickory County, MO\"\t29085\n\"Benton County, MO\"\t29015\t\"Morgan County, MO\"\t29141\n\"Benton County, MO\"\t29015\t\"Pettis County, MO\"\t29159\n\"Benton County, MO\"\t29015\t\"St. Clair County, MO\"\t29185\n\"Bollinger County, MO\"\t29017\t\"Bollinger County, MO\"\t29017\n\"Bollinger County, MO\"\t29017\t\"Cape Girardeau County, MO\"\t29031\n\"Bollinger County, MO\"\t29017\t\"Madison County, MO\"\t29123\n\"Bollinger County, MO\"\t29017\t\"Perry County, MO\"\t29157\n\"Bollinger County, MO\"\t29017\t\"Stoddard County, MO\"\t29207\n\"Bollinger County, 
